vi "Get Sensor Data.vi"(8 "error in":errorcluster, 11 "VisionServerRef in":T1) -> (0 "error out":errorcluster, 2 "Sensor":T2, 3 "VisionServerRef out":T1)   [LabVIEW 2016, in "Vision Server.lvclass"]
uses:
  Vision Server.lvclass
  typedef/Sensor Message JSON.ctl
  typedef/Vision Server Ref.ctl
  Vision Server.lvclass/Vision Server.ctl
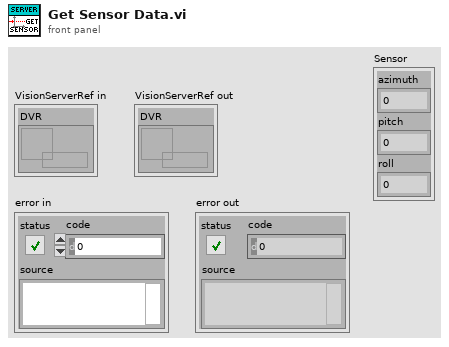
[diagram p1: front panel]
types:
  T1 = typedef "Vision Server.lvclass/Vision Server Ref.ctl" = cluster{"DVR":refnum<data-value>}
  T2 = typedef "Vision Server.lvclass/Sensor Message JSON.ctl" = cluster{"azimuth":dbl, "pitch":dbl, "roll":dbl}
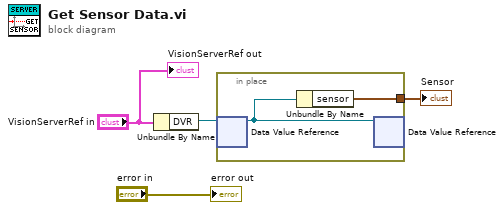
[diagram p0: block diagram]
diagram:
  n1 = Unbundle By Name("VisionServerRef in") -> ("DVR"=w3:refnum<data-value>)
  n2 = in-place {
    in-place-border: [w6] -> w4
    n3 = in-place-dvr #1(w3) -> (w5:refnum<class "Vision Server.lvclass">)  [unwired: 1 out]
    n4 = Unbundle By Name(w5) -> ("sensor"=w6:T2)
    n5 = in-place-dvr #1(w5) -> ()  [unwired: 2 out]
  }
  "Sensor" <- w4
  "error out" <- "error in"
  "VisionServerRef out" <- "VisionServerRef in"
